vi "adder.vi"(4 "covariance_nontarget":dbl[][](array[numeric]), 6 "covariance_target":dbl[][](array[numeric]), 8 "alk":ext[][](array[numeric]), 9 "u(t+1)":dbl[][](array[numeric]), 11 "beta(t+1)":ext[](array[numeric])) -> (3 "beta(t)":ext[](array[numeric]))   [LabVIEW 2013]
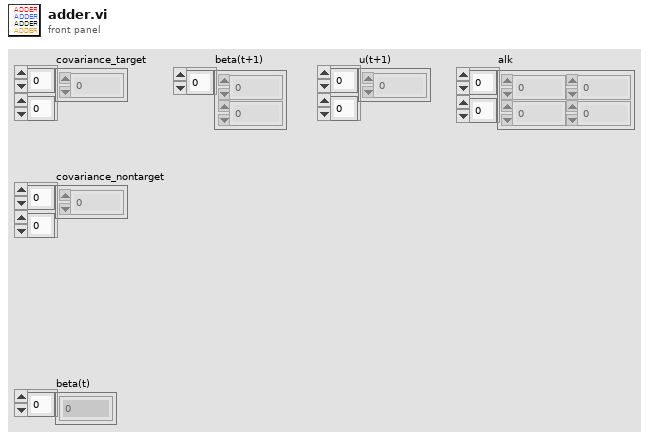
[diagram p1: front panel]
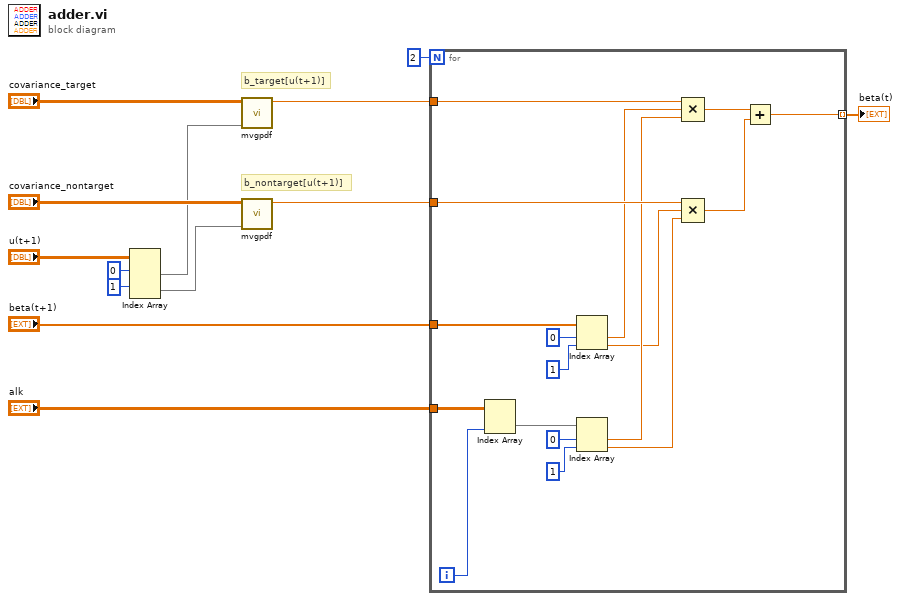
[diagram p0: block diagram]
diagram:
  # "b_nontarget[u(t+1)]"
  # "b_target[u(t+1)]"
  n1 = Index Array(array="u(t+1)", index (row) #1=0 ("index (row)"), index (row) #2=1 ("index (row)")) -> (element #1=w2:dbl[], element #2=w1:dbl[])  [unwired: 2 in]
  n2 = call "mvgpdf.vi"("input_ERP(normalized)"=w2, "covariance"="covariance_target") -> ("Gaussian_prob"=w10:ext)  [unwired: 9 in]
  n3 = call "mvgpdf.vi"("input_ERP(normalized)"=w1, "covariance"="covariance_nontarget") -> ("Gaussian_prob"=w9:ext)  [unwired: 9 in]
  n4 = for {
    N: 2 -> [_]
    tunnel: "beta(t+1)" -> [w29]
    tunnel: w10 -> [w23]
    tunnel: w9 -> [w22]
    tunnel: "alk" -> [w30]
    tunnel: [w15] -> w6 mode=indexing
    i -> [w14]
    n5 = Index Array(array=w30, index (col)=w14) -> (element=w24:ext[])  [unwired: 1 in]
    n6 = Index Array(array=w29, index #1=0 ("index"), index #2=1 ("index")) -> (element #1=w21:ext, element #2=w19:ext)
    n7 = Index Array(array=w24, index #1=0 ("index"), index #2=1 ("index")) -> (element #1=w20:ext, element #2=w18:ext)
    n8 = Compound Arithmetic op=MULTIPLY(w23, w21, w20) -> (w17:ext)
    n9 = Compound Arithmetic op=MULTIPLY(w22, w19, w18) -> (w16:ext)
    n10 = Add(x=w17, y=w16) -> (x+y=w15:ext)
  }
  "beta(t)" <- w6
